vi "rotate section.vi"(8 "To Facet":i32[][](array[numeric]), 9 "From Facet":i32[][](array[numeric]), 10 "From":i32[](array[numeric])=[1, 3, 4, 5], 11 "Enum":T1=enum."Right") -> (2 "To":cluster{"row":i32, "column":i32}[](array[cluster]), 3 "From":cluster{"row":i32, "column":i32}[](array[cluster]))   [LabVIEW 2019]
uses:
  section movement.ctl
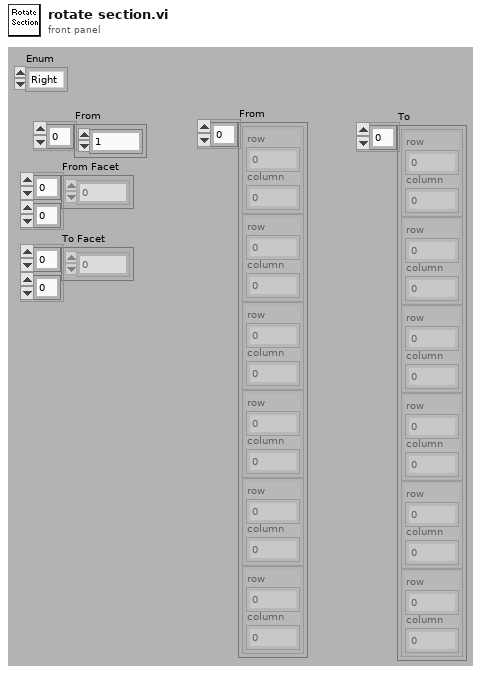
[diagram p1: front panel]
types:
  T1 = typedef "section movement.ctl" = enum16{"Left", "Right"}
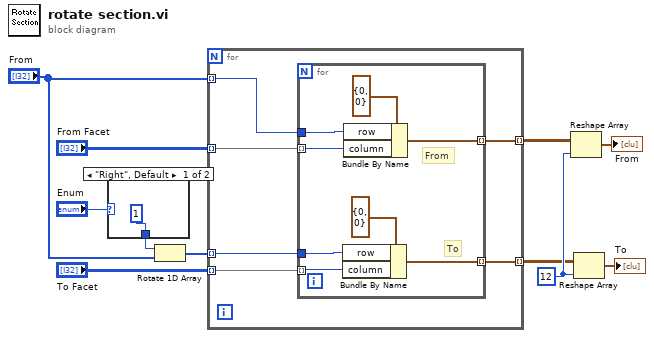
[diagram p0: block diagram]
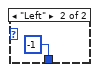
[diagram p2: hidden frame]
diagram:
  w11 = 12 ("dimension size")
  n1 = case shown="\"Right\", Default" "Enum" {
    tunnel: [1 -1] -> w3
    frame "Right", Default {
    }
    frame "Left" {
    }
  }
  n2 = Rotate 1D Array(1:"From", 2:w3) -> (0:w5:i32[])
  n3 = for {
    tunnel: w5 -> [w19] mode=indexing
    tunnel: "From" -> [w18] mode=indexing
    tunnel: [w17] -> w8 mode=indexing
    tunnel: [w16] -> w7 mode=indexing
    tunnel: "From Facet" -> [w15] mode=indexing
    tunnel: "To Facet" -> [w14] mode=indexing
    n4 = for {
      tunnel: w19 -> [w26]
      tunnel: w18 -> [w24]
      tunnel: [w23] -> w17 mode=indexing
      tunnel: [w22] -> w16 mode=indexing
      tunnel: w15 -> [w21] mode=indexing
      tunnel: w14 -> [w20] mode=indexing
      # "To"
      # "From"
      n5 = Bundle By Name(cluster=cluster{"row":i32, "column":i32} {"row"=0, "column"=0} ("From"), "row"=w26, "column"=w20) -> (w22:cluster{"row":i32, "column":i32})
      n6 = Bundle By Name(cluster=cluster{"row":i32, "column":i32} {"row"=0, "column"=0} ("From"), "row"=w24, "column"=w21) -> (w23:cluster{"row":i32, "column":i32})
    }
  }
  n7 = Reshape Array(w8, w11) -> (→"From":cluster{"row":i32, "column":i32}[])
  n8 = Reshape Array(w7, w11) -> (→"To":cluster{"row":i32, "column":i32}[])
